vi "AnalyzerSettingsFGV.vi"(8 "FGVAction (Read)":T7, 11 "AnalyzerSettingsIn":T1={"Create NS Timeout Code"=-314004, "Destroy NS Timeout Code"=-314004, "All threads"=[], "Connected to app?"=FALSE, "AnalysisSettings"={"Fault Thresholds"={"Parameters labels"=[], "Parameters thresholds"=[], "Freqs and thresholds"=[], "Orders and thresholds"=[]}, "Analysis series name"="Analiza", "Save data analysis?"=TRUE, "Band size"=20, "OrderAnalysis?"=TRUE, "Accelerometer"=enum."MMA7351", "fs [Hz]"=4000.0, "Pulse per revolution"=1}}) -> (3 "AnalyzerSettingsOut":T1={"Create NS Timeout Code"=-314004, "Destroy NS Timeout Code"=-314004, "All threads"=[], "Connected to app?"=FALSE, "AnalysisSettings"={"Fault Thresholds"={"Parameters labels"=[], "Parameters thresholds"=[], "Freqs and thresholds"=[], "Orders and thresholds"=[]}, "Analysis series name"="Analiza", "Save data analysis?"=TRUE, "Band size"=20, "OrderAnalysis?"=TRUE, "Accelerometer"=enum."MMA7351", "fs [Hz]"=4000.0, "Pulse per revolution"=1}})   [LabVIEW 2019]
uses:
  FGVAction.ctl
  AnalyzerSettings.ctl
  AmasterVIs/AThreads.ctl
  VibrationDiagnosisDesktopApp/mainVIs/DialogsVIs/AnalysisSettings.ctl
  analyzeAccelerationDataVIs/calculateFaultIndicatorsVIs/Thresholds.ctl
  analyzeAccelerationDataVIs/calculateFaultIndicatorsVIs/FaultParameter.ctl
  aquireAccelerationDataVIs/Accelerometer.ctl
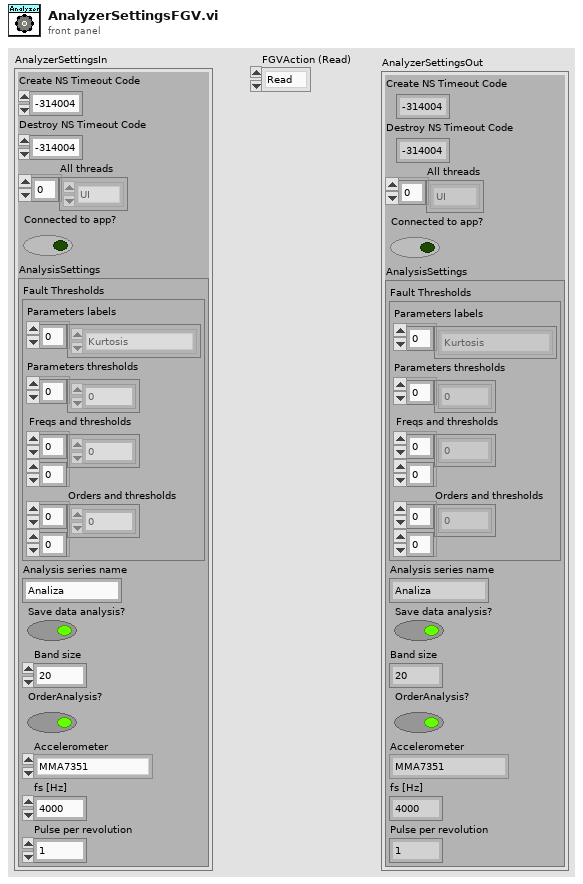
[diagram p1: front panel]
types:
  T1 = typedef "AnalyzerSettings.ctl" = cluster{"Create NS Timeout Code":i32, "Destroy NS Timeout Code":i32, "All threads":T2[], "Connected to app?":bool, "AnalysisSettings":T3}
  T2 = typedef "AThreads.ctl" = enum16{"UI", "analyzeAccelerationData", "aquireAccelerationData", "communicateWebServices", "TDMSmanager", "aquireTachoSignal"}
  T3 = typedef "AnalysisSettings.ctl" = cluster{"Fault Thresholds":T4, "Analysis series name":string, "Save data analysis?":bool, "Band size":i32, "OrderAnalysis?":bool, "Accelerometer":T6, "fs [Hz]":dbl, "Pulse per revolution":u16}
  T4 = typedef "Thresholds.ctl" = cluster{"Parameters labels":T5[], "Parameters thresholds":dbl[], "Freqs and thresholds":dbl[][], "Orders and thresholds":dbl[][]}
  T5 = typedef "FaultParameter.ctl" = enum16{"Kurtosis", "RMS", "Crest factor"}
  T6 = typedef "Accelerometer.ctl" = enum16{"None", "MPU6050", "MMA7351"}
  T7 = typedef "FGVAction.ctl" = enum16{"Read", "Write"}
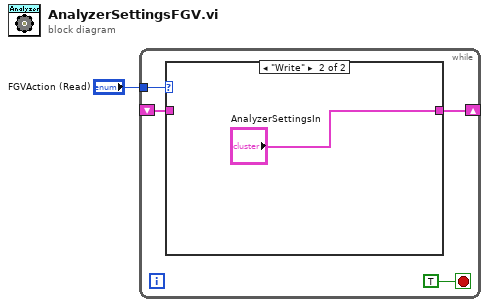
[diagram p0: block diagram]
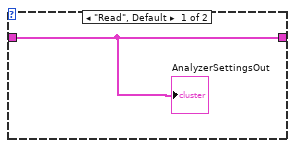
[diagram p2: hidden frame]
diagram:
  n1 = while {
    tunnel: "FGVAction (Read)" -> [w4]
    shift-right: [w2] -> _
    shift-left: _ -> [w3]
    stop <- TRUE stop-if-true
    n2 = case shown="\"Write\"" w4 {
      tunnel: w3 -> [w6 _]
      tunnel: [w6 "AnalyzerSettingsIn"] -> w2
      frame "Read", Default {
        "AnalyzerSettingsOut" <- w6
      }
      frame "Write" {
      }
    }
  }
